vi "TSP.vi"(0 "System no.":i32=1 min=1 max=4 step=1, 2 "Sensor to set":string[](array[string]), 3 "Sensor position":dbl[](array[numeric]) format="%.6f", 4 "No. of digits":i16=4, 5 "error in":errorcluster) -> (19 "error out":errorcluster)   [LabVIEW 2020]
doc: "Sets sensor position for the specified sensor number.\n\nMercury_GCS:"
panel:
  # "Sets sensor position for the specified sensor number."
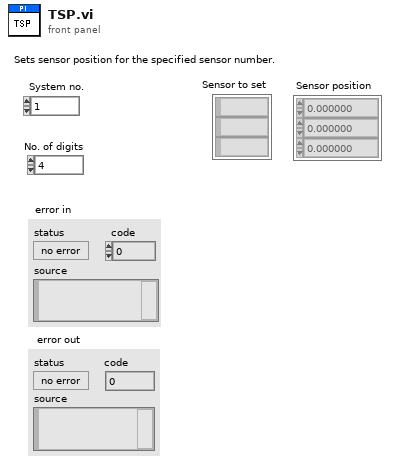
[diagram p1: front panel]
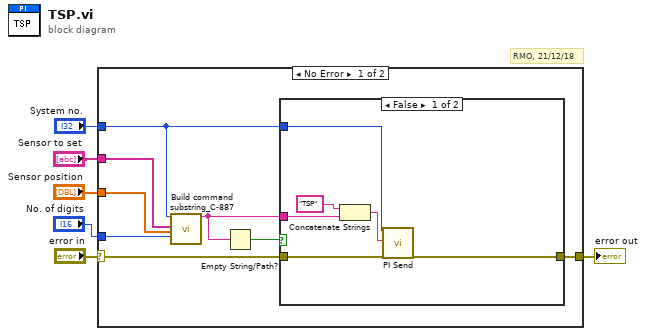
[diagram p0: block diagram]
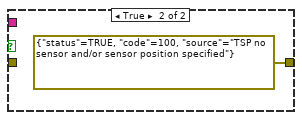
[diagram p2: hidden frame]
diagram:
  # "RMO, 21/12/18"
  n1 = case shown="No Error" "error in" {
    selector: "error in" -> [w9 w22]
    tunnel: "Sensor to set" -> [w10 _]
    tunnel: [w14 w22] -> w5
    tunnel: "System no." -> [w13 _]
    tunnel: "Sensor position" -> [w12 _]
    tunnel: "No. of digits" -> [w11 _]
    frame No Error {
      n2 = call "Build command substring_C-887.vi"("System no."=w13, "Affected axes"=w10, "Parameters"=w12, "No. of digits"=w11) -> ("Command substring"=w8:string)  [unwired: 3 in, 12 out]
      n3 = Empty String/Path?(string/path=w8) -> (empty?=w7:bool)
      n4 = case shown="False" w7 {
        tunnel: [w18 errorcluster {"status"=TRUE, "code"=100, "source"="TSP no sensor and/or sensor position specified"} ("error out")] -> w14
        tunnel: w13 -> [w17 _]
        tunnel: w8 -> [w16 _]
        tunnel: w9 -> [w15 _]
        frame False {
          n5 = Concatenate Strings("TSP", w16) -> (w20:string)
          n6 = call "PI Send.vi"("System no."=w17, "String to send"=w20, "error in"=w15) -> ("error out"=w18:errorcluster)  [unwired: 3 in, 13 out]
        }
        frame True {
        }
      }
    }
    frame Error {
    }
  }
  "error out" <- w5
